vi "Example IMAQdx Cam and XDisplay_temp.vi"() -> ()   [LabVIEW 2014]
uses:
  <vilib>/userdefined/High Color/IMAQdx.ctl
  XDisplay/POLARIS IMAQ Display.xctl
  IMAQdx Cam/IMAQdx Cam.lvclass
panel:
  in  "XDisplay":cluster{"Image":T1}(xcontrol)
  in  "stop":bool
  in  "Camera Name":T2="JustageCam"
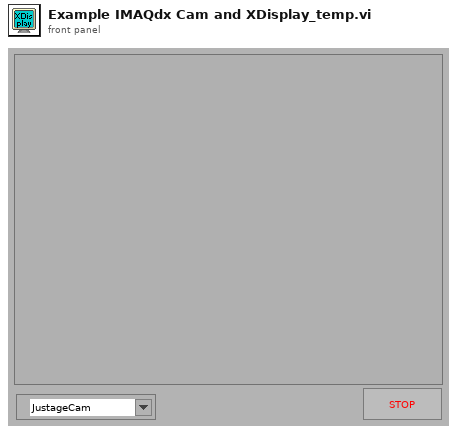
[diagram p1: front panel]
types:
  T1 = typedef "IMAQ Image.ctl" = refnum<image>
  T2 = typedef "IMAQdx.ctl" = refnum<k21>
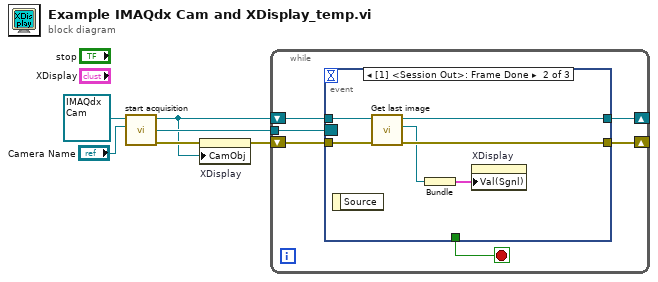
[diagram p0: block diagram]
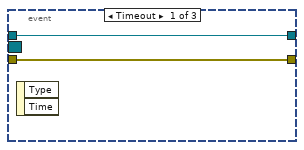
[diagram p2: hidden frame]
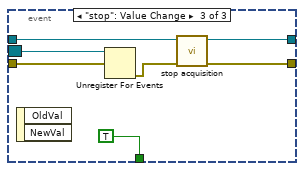
[diagram p3: hidden frame]
diagram:
  n1 = call-dynamic "start acquisition.vi"("Camera Name"="Camera Name", "IMAQdx Cam in"=refnum<class "IMAQdx Cam.lvclass"> refnum ("IMAQdx Cam.lvclass")) -> ("error out"=w3:errorcluster, "Event Registration Refnum"=w5:refnum<event-registration>, "IMAQdx Cam out"=w1:refnum<class "IMAQdx Cam.lvclass">)  [unwired: 7 in]
  n2 = property on="XDisplay" class="POLARIS IMAQ Display (strict)"(error in=w3, "CamObj"=w1) -> (error out=w2:errorcluster)  [unwired: 1 in, 1 out]
  n3 = while {
    tunnel: w5 -> [w7]
    shift-right: [w10] -> _
    shift-left: w1 -> [w12]
    shift-right: [w9] -> _
    shift-left: w2 -> [w11]
    stop <- w8 stop-if-true
    n4 = event shown="[1] <Session Out>: Frame Done" {
      selector: w7 -> [_ _ w26]
      dyn-events: _ -> [_ _ _]
      timeout: _ -> [_ _ _]
      tunnel: w12 -> [w13 w20 w24]
      tunnel: w11 -> [w14 w19 w25]
      tunnel: [w13 w18 w22] -> w10
      tunnel: [w14 w17 w21] -> w9
      tunnel: [_ _ TRUE] -> w8
      event Timeout {
        n5 = event-data() -> ()  [unwired: 1 in, 2 out]
      }
      event event #0x0 {
        n6 = event-data() -> ()  [unwired: 1 in, 1 out]
        n7 = call-dynamic "Get last image.vi"("error in (no error)"=w19, "IMAQdx Cam in"=w20) -> ("error out"=w17:errorcluster, "Image Out"=w16:T1, "IMAQdx Cam out"=w18:refnum<class "IMAQdx Cam.lvclass">)  [unwired: 7 in]
        n8 = Bundle("Image Out"=w16) -> (w15:cluster{"Image Out":T1})  [unwired: 1 in]
        n9 = property on="XDisplay" class="POLARIS IMAQ Display (strict)"("Val(Sgnl)"=w15) -> ()  [unwired: 2 in, 2 out]
      }
      event "stop": Value Change {
        n10 = event-data() -> ()  [unwired: 1 in, 2 out]
        n11 = Unregister For Events(event registration refnum=w26, error in=w25) -> (error out=w23:errorcluster)
        n12 = call-dynamic "stop acquisition.vi"("error in (no error)"=w23, "IMAQdx Cam in"=w24) -> ("error out"=w21:errorcluster, "IMAQdx Cam out"=w22:refnum<class "IMAQdx Cam.lvclass">)  [unwired: 8 in]
      }
    }
  }
